vi "MSEncoder SubVI WfmCodeGen_PhaseScanII.vi"(6 "dm":ext, 7 "Stepwise":i32, 8 "f2":ext, 9 "m1":ext, 10 "f1":ext, 11 "MSEncoder.lvclass":refnum<class "MSEncoder.lvclass">) -> (0 "WfmCode":u64[](array[numeric]), 1 "RF status":T1, 2 "Scan time":dbl, 3 "mzTable":cluster{"t":dbl[], "mz":dbl[], "beta":dbl[]}, 4 "error out":errorcluster)   [LabVIEW 2018, in "MSEncoder.lvclass"]
uses:
  MSEncoder.lvclass
  MSEncoder.lvclass/MSEncoder.ctl
panel:
  in  "High Res":bool
  in  "Interrupt":bool
  out "Phase Scan II":cluster{"Scan time":ext, "Actual Freq":dbl}[](graph)
  out "Progress":dbl(slide) scale=0.0..322212.04607678554
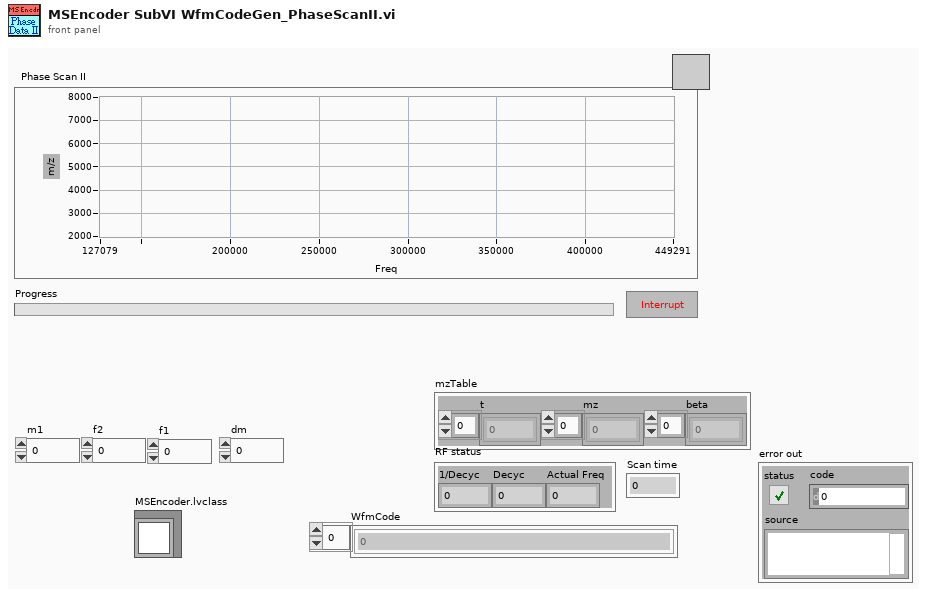
[diagram p1: front panel]
types:
  T1 = cluster{"1/Decyc":u32, "Decyc":u64, "Actual Freq":dbl}
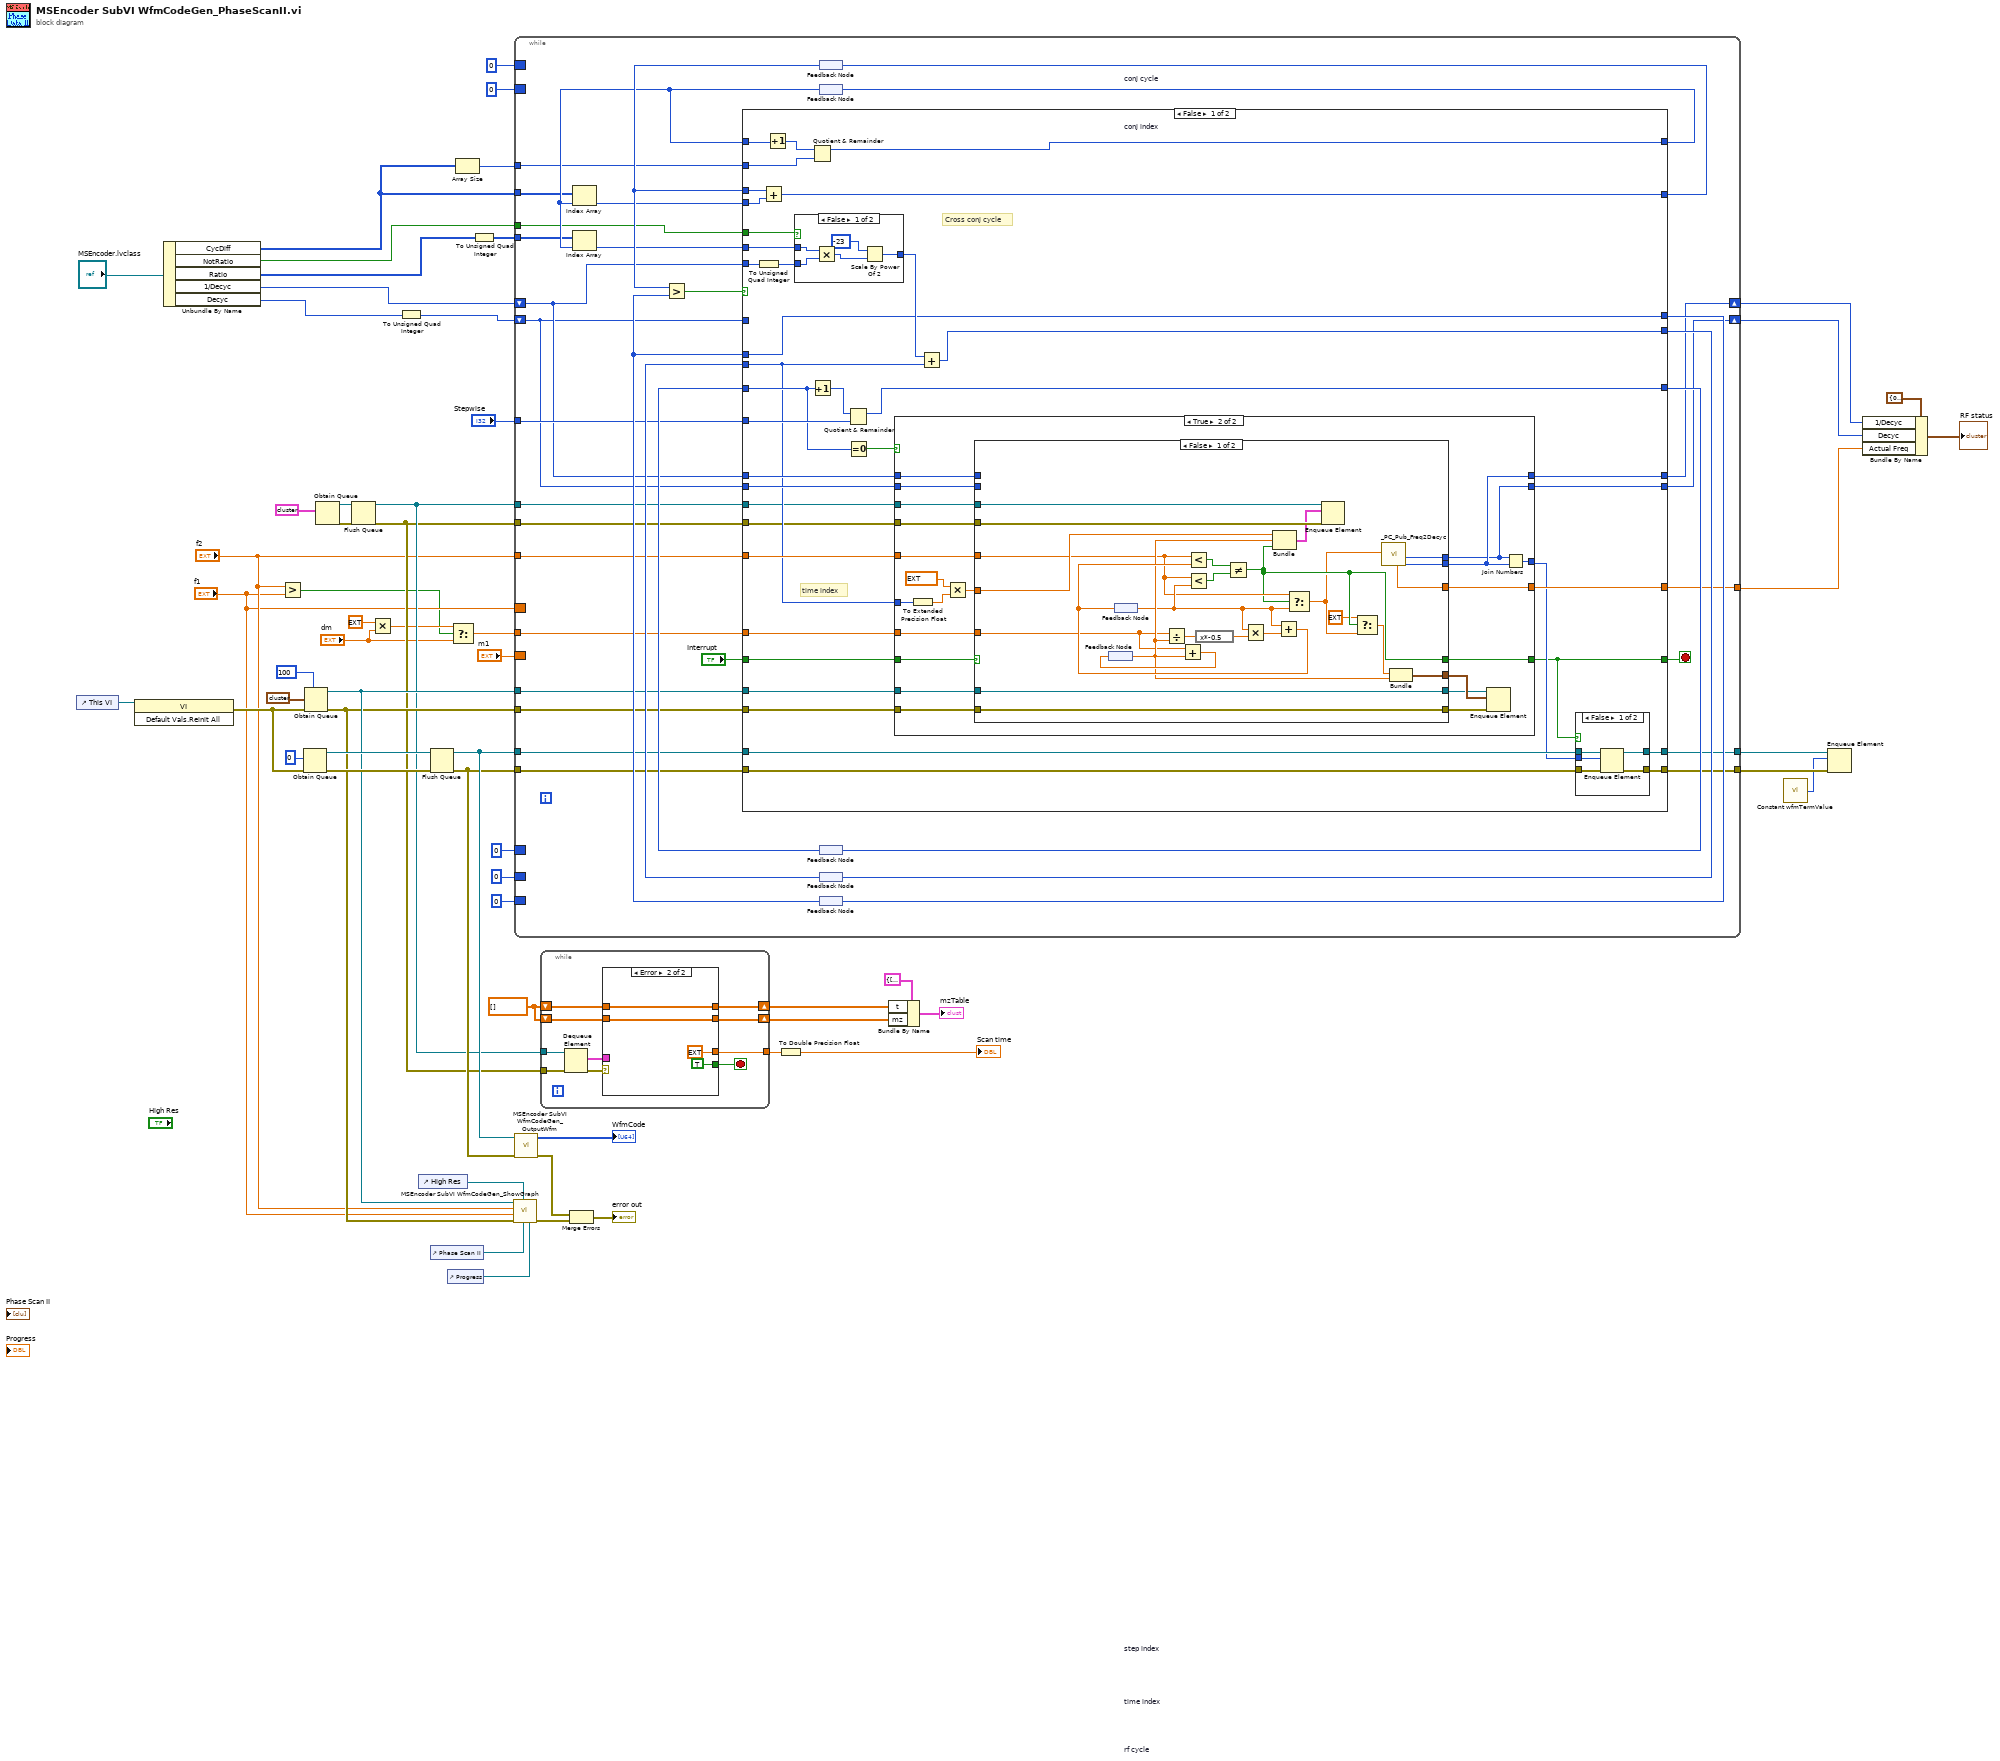
[diagram p0: block diagram]
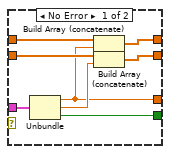
[diagram p2: hidden frame]
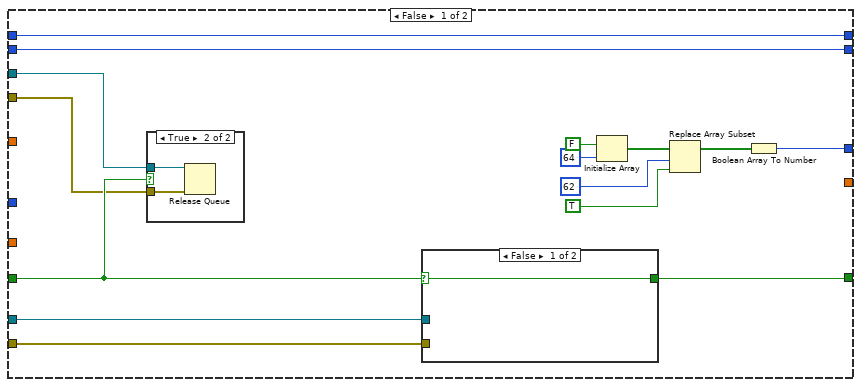
[diagram p5: hidden frame]
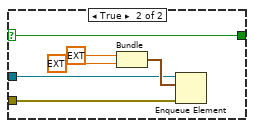
[diagram p7: hidden frame]
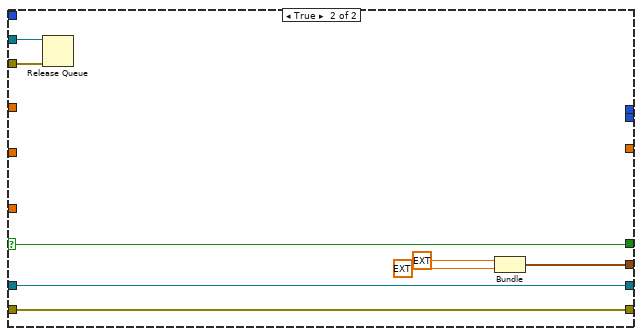
[diagram p8: hidden frame]
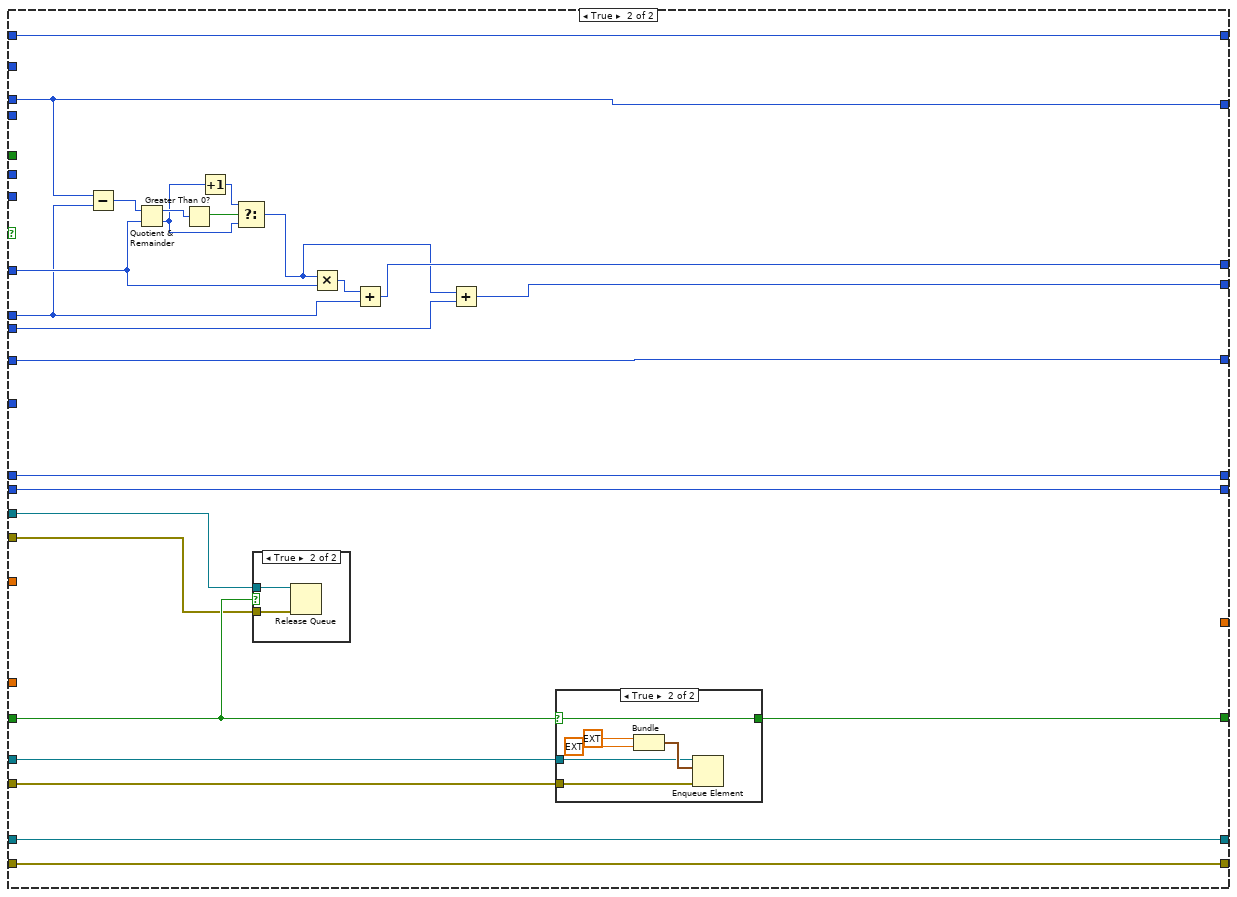
[diagram p9: hidden frame]
diagram:
  w1 = ext[] []
  n1 = control-ref of="This VI"() -> (w28:refnum<vi>)
  n2 = invoke class="VI" method="Default Vals.Reinit All"(reference=w28) -> (error out=w27:errorcluster)  [unwired: 2 in, 2 out]
  n3 = Unbundle By Name("MSEncoder.lvclass") -> ("CycDiff"=w48:u64[], "NotRatio"=w47:bool, "Ratio"=w58:u16[], "1/Decyc"=w54:u32, "Decyc"=w53:u32)
  n4 = Greater?(x="f2", y="f1") -> (0:w6:bool)
  n5 = Obtain Queue(element data type=u64 0, error in (no error)=w27) -> (queue out=w43:refnum<queue>, error out=w44:errorcluster)  [unwired: 3 in, 1 out]
  n6 = Obtain Queue(max queue size (-1, unlimited)=100, element data type=cluster{"Scan time":ext, "Actual Freq":ext} {"Scan time"=0.0, "Actual Freq"=0.0} ("output cluster"), error in (no error)=w27) -> (queue out=w36:refnum<queue>, error out=w35:errorcluster)  [unwired: 2 in, 1 out]
  n7 = Obtain Queue(element data type=cluster{ext, "m1":ext, bool} {0.0, "m1"=0.0, FALSE} ("output cluster")) -> (queue out=w26:refnum<queue>, error out=w25:errorcluster)  [unwired: 4 in, 1 out]
  n8 = Flush Queue(queue=w26, error in (no error)=w25) -> (queue out=w23:refnum<queue>, error out=w22:errorcluster)  [unwired: 1 out]
  n9 = Multiply(x=ext -1.0, y="dm") -> (x*y=w7:ext)
  n10 = To Unsigned Quad Integer(1:w53) -> (0:w49:u64)
  n11 = control-ref of="High Res"() -> (w3:refnum<vi>)
  n12 = Flush Queue(queue=w43, error in (no error)=w44) -> (queue out=w39:refnum<queue>, error out=w38:errorcluster)  [unwired: 1 out]
  n13 = control-ref of="Phase Scan II"() -> (w34:refnum<vi>)
  n14 = control-ref of="Progress"() -> (w33:refnum<vi>)
  n15 = Select(t=w7, s=w6, f="dm") -> (s? t:f=w4:ext)
  n16 = Array Size(array=w48) -> (size(s)=w60:i32)
  n17 = To Unsigned Quad Integer(1:w58) -> (0:w50:u64[])
  n18 = call "MSEncoder SubVI WfmCodeGen_ShowGraph.vi"("progress refnum"=w33, "system graph refnum"=w34, "Graph Display"=w3, "error in (no error)"=w35, "X Scale.Range:Minimun"="f1", "X Scale.Range:Maximum"="f2", "Display queue in"=w36) -> ("error out"=w31:errorcluster)  [unwired: 4 in]
  n19 = while {
    tunnel: w48 -> [w92]
    tunnel: "Stepwise" -> [w82]
    border: u64 0 -> [_]
    border: u64 0 -> [_]
    tunnel: w60 -> [w88]
    border: u64 0 -> [_]
    shift-right: [w76] -> w14
    shift-left: w49 -> [w78]
    shift-right: [w77] -> w13
    shift-left: w54 -> [w79]
    tunnel: w50 -> [w91]
    tunnel: "f2" -> [w80]
    tunnel: w36 -> [w74]
    tunnel: w35 -> [w73]
    border: 0 -> [_]
    border: 0 -> [_]
    tunnel: [w72] -> w15
    tunnel: w47 -> [w70]
    tunnel: w39 -> [w69]
    tunnel: w38 -> [w68]
    tunnel: [w67] -> w42
    tunnel: [w66] -> w41
    border: "f1" -> [_]
    border: "m1" -> [_]
    tunnel: w23 -> [w64]
    tunnel: w22 -> [w63]
    tunnel: w4 -> [w62]
    stop <- w75 stop-if-true
    n20 = feedback #1 "conj cycle"() -> (w96:u64)
    n21 = feedback #2 "conj index"() -> (w93:i32)
    n22 = Index Array(array=w92, index=w93) -> (element=w89:u64)
    n23 = Index Array(array=w91, index=w93) -> (element=w90:u64)
    n24 = feedback #3 "step index"() -> (w94:i32)
    n25 = feedback #4 "time index"() -> (w84:u64)
    n26 = feedback #5 "rf cycle"() -> (w95:u64)
    n27 = Greater?(x=w96, y=w95) -> (0:w71:bool)
    n28 = case shown="False" w71 {
      tunnel: w90 -> [w128 _]
      tunnel: w89 -> [w134 _]
      tunnel: w96 -> [w133 w241]
      tunnel: w78 -> [_ w240]
      tunnel: w95 -> [w108 w239]
      tunnel: w88 -> [w130 _]
      tunnel: [w132 w241] -> w87
      tunnel: w79 -> [w127 _]
      tunnel: w93 -> [w123 w250]
      tunnel: [w129 w250] -> w86
      tunnel: [w121 w246] -> w85
      tunnel: w84 -> [w110 w249]
      tunnel: [w108 w247] -> w83
      tunnel: w82 -> [w126 _]
      tunnel: [w125 w243] -> w81
      tunnel: w94 -> [w124 w243]
      tunnel: w80 -> [w122 _]
      tunnel: w79 -> [w120 w245]
      tunnel: w78 -> [w119 w244]
      tunnel: [w118 w245] -> w77
      tunnel: [w117 w244] -> w76
      tunnel: [w100 w231] -> w75
      tunnel: w74 -> [w116 w230]
      tunnel: w73 -> [w115 w229]
      tunnel: [w114 _] -> w72
      tunnel: w70 -> [w107 _]
      tunnel: w69 -> [w106 w233]
      tunnel: w68 -> [w105 w232]
      tunnel: [w103 w233] -> w67
      tunnel: [w102 w232] -> w66
      tunnel: "Interrupt" -> [w101 w228]
      tunnel: w64 -> [w99 w227]
      tunnel: w63 -> [w98 w226]
      tunnel: w62 -> [w97 _]
      frame False {
        # "time index"
        # "Cross conj cycle"
        n29 = To Unsigned Quad Integer(1:w127) -> (0:w113:u64)
        n30 = Add(x=w133, y=w134) -> (x+y=w132:u64)
        n31 = Increment(x=w123) -> (x+1=w131:i32)
        n32 = case shown="False" w107 {
          tunnel: w128 -> [w144 w147]
          tunnel: w113 -> [w142 _]
          tunnel: [w143 w147] -> w109
          frame False {
            n33 = Multiply(x=w144, y=w142) -> (x*y=w146:u64)
            n34 = Scale By Power Of 2(n=i16 -23, x=w146) -> (x*2^n=w143:u64)
          }
          frame True {
          }
        }
        n35 = Quotient & Remainder(x=w131, y=w130) -> (x-y*floor(x/y)=w129:i32)  [unwired: 1 out]
        n36 = Increment(x=w124) -> (x+1=w112:i32)
        n37 = Quotient & Remainder(x=w112, y=w126) -> (x-y*floor(x/y)=w125:i32)  [unwired: 1 out]
        n38 = Equal To 0?(x=w124) -> (x = 0?=w111:bool)
        n39 = case shown="True" w111 {
          tunnel: w122 -> [_ w192]
          tunnel: [w156 w191] -> w104
          tunnel: w110 -> [_ w188]
          tunnel: [w154 w184] -> w118
          tunnel: [w155 w183] -> w117
          tunnel: w120 -> [w154 w174]
          tunnel: w119 -> [w155 w173]
          tunnel: [w153 w182] -> w100
          tunnel: w116 -> [w152 w179]
          tunnel: w115 -> [w151 w177]
          tunnel: [_ w185] -> w114
          tunnel: w101 -> [w150 w181]
          tunnel: w99 -> [w149 w176]
          tunnel: w98 -> [w148 w175]
          tunnel: w97 -> [_ w172]
          frame False {
            n40 = case shown="True" w150 {
              tunnel: w149 -> [_ w164]
              tunnel: w148 -> [_ w163]
              frame False {
              }
              frame True {
                n41 = Release Queue(queue=w164, error in (no error)=w163) -> ()  [unwired: 1 in, 3 out]
              }
            }
            n42 = case shown="False" w150 {
              selector: w150 -> [w165 w166]
              tunnel: w152 -> [_ w168]
              tunnel: w151 -> [_ w167]
              tunnel: [w165 w166] -> w153
              frame False {
              }
              frame True {
                n43 = Bundle(ext -1.0, ext 0.0) -> (w171:cluster{ext, ext})  [unwired: 1 in]
                n44 = Enqueue Element(queue=w168, element=w171, error in (no error)=w167) -> ()  [unwired: 1 in, 3 out]
              }
            }
            n45 = Initialize Array(FALSE, 64 ("dimension size")) -> (w160:bool[])
            n46 = Replace Array Subset(array=w160, new element=TRUE, index=62) -> (w157:bool[])
            n47 = Boolean Array To Number(Boolean array=w157) -> (number=w156:u64)
          }
          frame True {
            n48 = To Extended Precision Float(1:w188) -> (0:w189:ext)
            n49 = Multiply(x=ext 2.5e-08, y=w189) -> (x*y=w187:ext)
            n50 = case shown="False" w181 {
              selector: w181 -> [_ w225]
              tunnel: w192 -> [w198 _]
              tunnel: w187 -> [w200 _]
              tunnel: [w217 w222] -> w186
              tunnel: [w216 _] -> w185
              tunnel: [w215 _] -> w184
              tunnel: [w214 _] -> w183
              tunnel: [w196 w225] -> w182
              tunnel: [w213 w221] -> w180
              tunnel: w179 -> [w213 w221]
              tunnel: [w212 w220] -> w178
              tunnel: w177 -> [w212 w220]
              tunnel: w176 -> [w207 w219]
              tunnel: w175 -> [w206 w218]
              tunnel: w174 -> [_ _]
              tunnel: w173 -> [_ _]
              tunnel: w172 -> [w197 _]
              frame False {
                n51 = feedback #6() -> (w201:ext)
                n52 = feedback #7() -> (w199:ext)
                n53 = Divide(x=w197, y=w201) -> (x/y=w211:ext)
                n54 = Add(x=w197, y=w201) -> (x+y=w208:ext)
                n55 = feedback-in #6(w208) -> ()
                n56 = Less?(x=w198, y=w199) -> (x < y?=w202:bool)
                n57 = expression code="x*-0.5"(w211) -> (w210:ext)
                n58 = Multiply(x=w199, y=w210) -> (x*y=w209:ext)
                n59 = Add(x=w199, y=w209) -> (x+y=w204:ext)
                n60 = feedback-in #7(w204) -> ()
                n61 = Less?(x=w198, y=w204) -> (x < y?=w203:bool)
                n62 = Not Equal?(x=w203, y=w202) -> (x != y?=w196:bool)
                n63 = Bundle(w200, "m1"=w201, w196) -> (w205:cluster{ext, "m1":ext, bool})  [unwired: 1 in]
                n64 = Select(t=w198, s=w196, f=w199) -> (s? t:f=w195:ext)
                n65 = Enqueue Element(queue=w207, element=w205, error in (no error)=w206) -> ()  [unwired: 1 in, 3 out]
                n66 = Select(t=ext -2.0, s=w196, f=w195) -> (s? t:f=w193:ext)
                n67 = call "_PC_Pub_Freq2Decyc.vi"("Freq"=w195) -> ("(1/Decyc)*2^8"=w215:u32, "Decyc*2^32"=w214:u32, "Actual Freq"=w216:dbl)  [unwired: 4 in, 2 out]
                n68 = Bundle("f1"=w193, "m1"=w201) -> (w217:cluster{"f1":ext, "m1":ext})  [unwired: 1 in]
              }
              frame True {
                n69 = Release Queue(queue=w219, error in (no error)=w218) -> ()  [unwired: 1 in, 3 out]
                n70 = Bundle(ext -1.0, ext 0.0) -> (w222:cluster{ext, ext})  [unwired: 1 in]
              }
            }
            n71 = Enqueue Element(queue=w180, element=w186, error in (no error)=w178) -> ()  [unwired: 1 in, 3 out]
            n72 = Join Numbers(hi=w183, lo=w184) -> ((hi.lo)=w191:u64)
          }
        }
        n73 = Add(x=w109, y=w110) -> (x+y=w121:u64)
        n74 = case shown="False" w100 {
          tunnel: w106 -> [w139 w141]
          tunnel: w105 -> [w138 w140]
          tunnel: w104 -> [w137 _]
          tunnel: [w136 w141] -> w103
          tunnel: [w135 w140] -> w102
          frame False {
            n75 = Enqueue Element(queue=w139, element=w137, error in (no error)=w138) -> (queue out=w136:refnum<queue>, error out=w135:errorcluster)  [unwired: 1 in, 1 out]
          }
          frame True {
          }
        }
      }
      frame True {
        n76 = Subtract(x=w241, y=w239) -> (x-y=w242:u64)
        n77 = Quotient & Remainder(x=w242, y=w240) -> (x-y*floor(x/y)=w238:u64, floor(x/y)=w235:u64)
        n78 = Greater Than 0?(x=w238) -> (x > 0?=w237:bool)
        n79 = Increment(x=w235) -> (x+1=w236:u64)
        n80 = Select(t=w236, s=w237, f=w235) -> (s? t:f=w234:u64)
        n81 = case shown="True" w228 {
          tunnel: w227 -> [_ w252]
          tunnel: w226 -> [_ w251]
          frame False {
          }
          frame True {
            n82 = Release Queue(queue=w252, error in (no error)=w251) -> ()  [unwired: 1 in, 3 out]
          }
        }
        n83 = Multiply(x=w234, y=w240) -> (x*y=w248:u64)
        n84 = Add(x=w248, y=w239) -> (x+y=w247:u64)
        n85 = Add(x=w234, y=w249) -> (x+y=w246:u64)
        n86 = case shown="True" w228 {
          selector: w228 -> [w253 w254]
          tunnel: w230 -> [_ w256]
          tunnel: w229 -> [_ w255]
          tunnel: [w253 w254] -> w231
          frame False {
          }
          frame True {
            n87 = Bundle(ext -1.0, ext 0.0) -> (w259:cluster{ext, ext})  [unwired: 1 in]
            n88 = Enqueue Element(queue=w256, element=w259, error in (no error)=w255) -> ()  [unwired: 1 in, 3 out]
          }
        }
      }
    }
    n89 = feedback-in #1(w87) -> ()
    n90 = feedback-in #2(w86) -> ()
    n91 = feedback-in #3(w81) -> ()
    n92 = feedback-in #4(w85) -> ()
    n93 = feedback-in #5(w83) -> ()
  }
  n94 = call "MSEncoder SubVI WfmCodeGen_OutputWfm.vi"("error in (no error)"=w38, "calc wfm queue"=w39) -> ("error out"=w32:errorcluster, "WfmCode"=→"WfmCode":u64[])  [unwired: 8 in]
  n95 = while {
    tunnel: w23 -> [w269]
    tunnel: w22 -> [w268]
    shift-right: [w266] -> w20
    shift-left: w1 -> [w263]
    shift-right: [w265] -> w2
    shift-left: w1 -> [w264]
    tunnel: [w262] -> w18
    stop <- w260 stop-if-true
    n96 = Dequeue Element(queue=w269, error in (no error)=w268) -> (element=w267:cluster{ext, "m1":ext, bool}, error out=w261:errorcluster)  [unwired: 1 in, 2 out]
    n97 = case shown="Error" w261 {
      tunnel: w267 -> [w277 _]
      tunnel: [w275 w281] -> w266
      tunnel: [w274 w280] -> w265
      tunnel: w264 -> [w273 w280]
      tunnel: w263 -> [w272 w281]
      tunnel: [w271 ext 0.0] -> w262
      tunnel: [w270 TRUE] -> w260
      frame No Error {
        n98 = Unbundle(w277) -> (w271:ext, "m1"=w276:ext, w270:bool)
        n99 = Build Array (concatenate)(w272, w271) -> (w275:ext[])
        n100 = Build Array (concatenate)(w273, w276) -> (w274:ext[])
      }
      frame Error {
      }
    }
  }
  n101 = Merge Errors(w32, w31) -> (→"error out":errorcluster)
  n102 = To Double Precision Float(number=w18) -> (double precision float=→"Scan time":dbl)
  n103 = Bundle By Name(cluster=cluster{"t":dbl[], "mz":dbl[], "beta":dbl[]} {"t"=[], "mz"=[], "beta"=[]} ("mzTable"), "t"=w20, "mz"=w2) -> (→"mzTable":cluster{"t":dbl[], "mz":dbl[], "beta":dbl[]})
  n104 = call "Constant wfmTermValue.vi"() -> ("wfm end value"=w40:u64)
  n105 = Enqueue Element(queue=w42, element=w40, error in (no error)=w41) -> ()  [unwired: 1 in, 3 out]
  n106 = Bundle By Name(cluster=T1 {"1/Decyc"=0, "Decyc"=0, "Actual Freq"=0.0} ("RF status"), "1/Decyc"=w13, "Decyc"=w14, "Actual Freq"=w15) -> (→"RF status":T1)
